vi "Do State N Times.vi"(10 "dimension size":i32, 11 "State":string) -> (3 "N Time State":string)   [LabVIEW 2013]
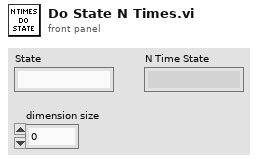
[diagram p1: front panel]
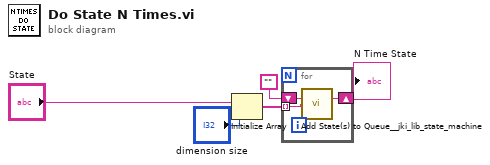
[diagram p0: block diagram]
diagram:
  n1 = Initialize Array("State", "dimension size") -> (w3:string[])
  n2 = for {
    tunnel: w3 -> [w8] mode=indexing
    shift-right: [w7] -> w5
    shift-left: "" -> [w6]
    n3 = call <vilib>:"Add State(s) to Queue__jki_lib_state_machine.vi"("State(s) in (\"\")"=w6, "State(s) at Back (\"\")"=w8) -> ("States Out"=w7:string)  [unwired: 13 in]
  }
  "N Time State" <- w5
